vi "Rolling Average.vi"(2 "Smooth Pts":i32, 7 "Input":dbl) -> (8 "Output":dbl)   [LabVIEW 2020]
uses:
  <vilib>/Analysis/baseanly.llb/Mean (DBL).vi
  <vilib>/Analysis/NI_AALBase.lvlib
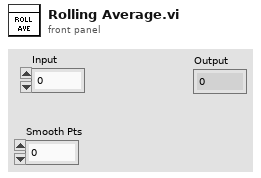
[diagram p1: front panel]
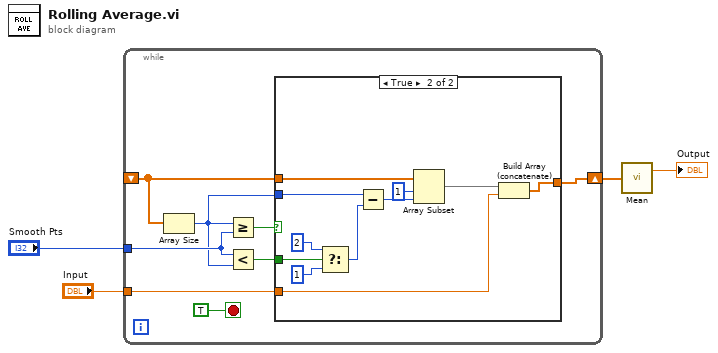
[diagram p0: block diagram]
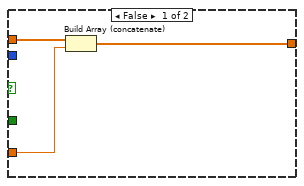
[diagram p2: hidden frame]
diagram:
  n1 = while {
    shift-right: [w9] -> w2
    shift-left: _ -> [w8]
    tunnel: "Input" -> [w10]
    tunnel: "Smooth Pts" -> [w7]
    stop <- TRUE stop-if-true
    n2 = Array Size(array=w8) -> (size(s)=w6:i32)
    n3 = Greater Or Equal?(x=w6, y=w7) -> (x >= y?=w11:bool)
    n4 = Less?(x=w7, y=w6) -> (x < y?=w5:bool)
    n5 = case shown="True" w11 {
      tunnel: w10 -> [w15 w23]
      tunnel: [w14 w22] -> w9
      tunnel: w8 -> [w13 w26]
      tunnel: w6 -> [_ w20]
      tunnel: w5 -> [_ w21]
      frame False {
        n6 = Build Array (concatenate)(w13, w15) -> (w14:dbl[])
      }
      frame True {
        n7 = Select(t=2, s=w21, f=1) -> (s? t:f=w16:i32)
        n8 = Subtract(x=w20, y=w16) -> (x-y=w19:i32)
        n9 = Array Subset(array=w26, index=1, length=w19) -> (w24:dbl[])
        n10 = Build Array (concatenate)(w24, w23) -> (w22:dbl[])
      }
    }
  }
  n11 = call-poly <vilib>:"Mean.vi"("X"=w2) -> ("mean"=→"Output":dbl)  [unwired: 1 out]
